vi "dfd_PR Cosine-Modulated Objective Function.vi"(3 "output control":T1, 4 "data":variant, 5 "X":dbl[](array[numeric])) -> (0 "error out":errorcluster, 1 "gradient":dbl[](array[numeric]), 2 "objective function value":dbl)   [LabVIEW 2017, in "NI_DigFilter_FilterBank.lvlib"]
uses:
  <vilib>/addons/Digital Filter Design/NI_DigFilter_FilterBank.lvlib
  <vilib>/Analysis/baseanly.llb/A x Vector.vi
  <vilib>/Analysis/baseanly.llb/Real Dot Product.vi
  <vilib>/Analysis/NI_AALBase.lvlib
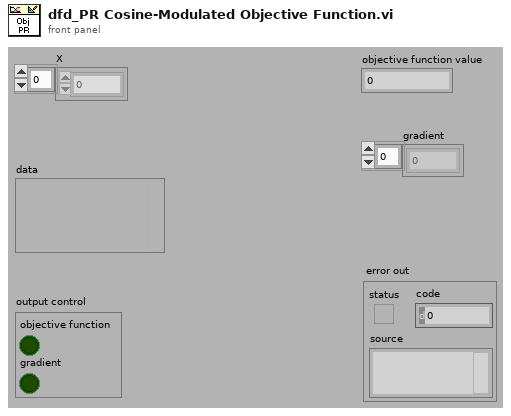
[diagram p1: front panel]
types:
  T1 = cluster{"objective function":bool, "gradient":bool}
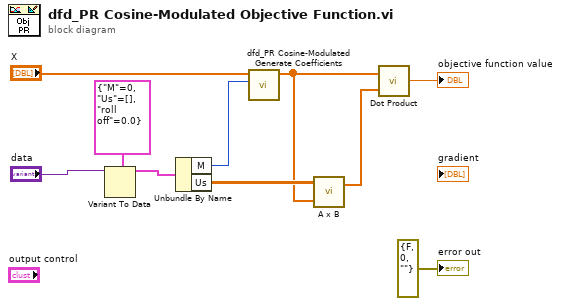
[diagram p0: block diagram]
diagram:
  n1 = Variant To Data(type=cluster{"M":i32, "Us":dbl[][], "roll off":dbl} {"M"=0, "Us"=[], "roll off"=0.0} ("output cluster"), Variant="data") -> (data=w8:cluster{"M":i32, "Us":dbl[][], "roll off":dbl})  [unwired: 1 in, 1 out]
  n2 = Unbundle By Name(w8) -> ("M"=w2:i32, "Us"=w6:dbl[][])
  n3 = call <vilib>:"dfd_PR Cosine-Modulated Generate Coefficients.vi"("M"=w2, "phi"="X") -> ("p"=w5:dbl[])  [unwired: 9 in]
  n4 = call-poly <vilib>:"A x B.vi"("Vector"=w5, "A"=w6) -> ("A x Vector"=w1:dbl[])  [unwired: 1 out]
  n5 = call-poly <vilib>:"Dot Product.vi"("Y Vector"=w1, "X Vector"=w5) -> ("X * Y"=→"objective function value":dbl)  [unwired: 1 out]
  "error out" <- errorcluster {"status"=FALSE, "code"=0, "source"=""} ("error out")
